vi "Initialize.vi"(8 "error in (no error)":errorcluster, 11 "Function in":refnum<class "Function.lvclass">) -> (0 "error out":errorcluster, 3 "Function out":refnum<class "Function.lvclass">)   [LabVIEW 2016, in "Function Actor.lvlib" / "Function.lvclass"]
doc: "Override configure.vi to setup any parameters for a function before acquiring.\n\nConfigure.vi is called by the 'Initialize Function Actor Core.vi,' which executes before Actor Core of the root function class. The root configure method populates the basic Function UI with information such as the hardware device in use and the name of the function. The base configure method calls 'Acquire.vi' once execution is complete. If beginning a recurring acquisition, it reset the iteration count to zero."
uses:
  <userlib>/Common Components/Function Actor/Function.lvclass
  C:/Program Files (x86)/National Instruments/LabVIEW 2016/vi.lib/ActorFramework/Actor/Actor.lvclass
  <vilib>/ActorFramework/Actor/Actor.lvclass/Actor.ctl
  <vilib>/ActorFramework/Message Enqueuer/Message Enqueuer.lvclass/Message Enqueuer.ctl
  <userlib>/Common Components/Function Actor/Function.lvclass/Function.ctl
  <userlib>/Common Components/Function Messages/Log in MsgList Msg/Log in MsgList Msg.lvclass/Log in MsgList Msg.ctl
  <vilib>/ActorFramework/Message Enqueuer/Init from Existing Queue.vi
  <vilib>/ActorFramework/Message Enqueuer/Enqueue.vi
  <userlib>/Common Components/Function Messages/TCP Connect Msg/TCP Connect Msg.lvclass
  C:/Program Files (x86)/National Instruments/LabVIEW 2016/vi.lib/ActorFramework/Message/Message.lvclass
  <userlib>/Common Components/Function Messages/WebSocket Handshake Msg/WebSocket Handshake Msg.lvclass
  <userlib>/Common Components/Function Messages/Log in MsgList Msg/Log in MsgList Msg.lvclass
  <userlib>/Common Components/Function Actor/Messages/Acquire Msg/Core Iterate Msg.lvclass
  <vilib>/ActorFramework/Message Priority Queue/Priority Enqueue.vi
  <vilib>/ActorFramework/Message Enqueuer/Message Enqueuer.lvclass
  <userlib>/Common Components/Hardware/Abstract Hardware/Hardware.lvclass
  <vilib>/ActorFramework/Actor/Actor.lvclass
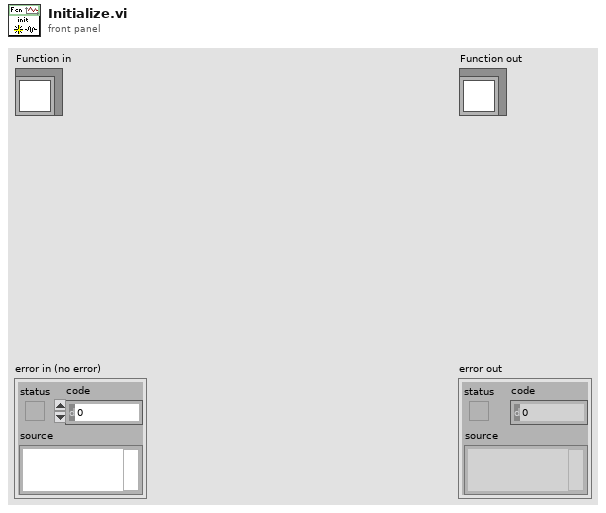
[diagram p1: front panel]
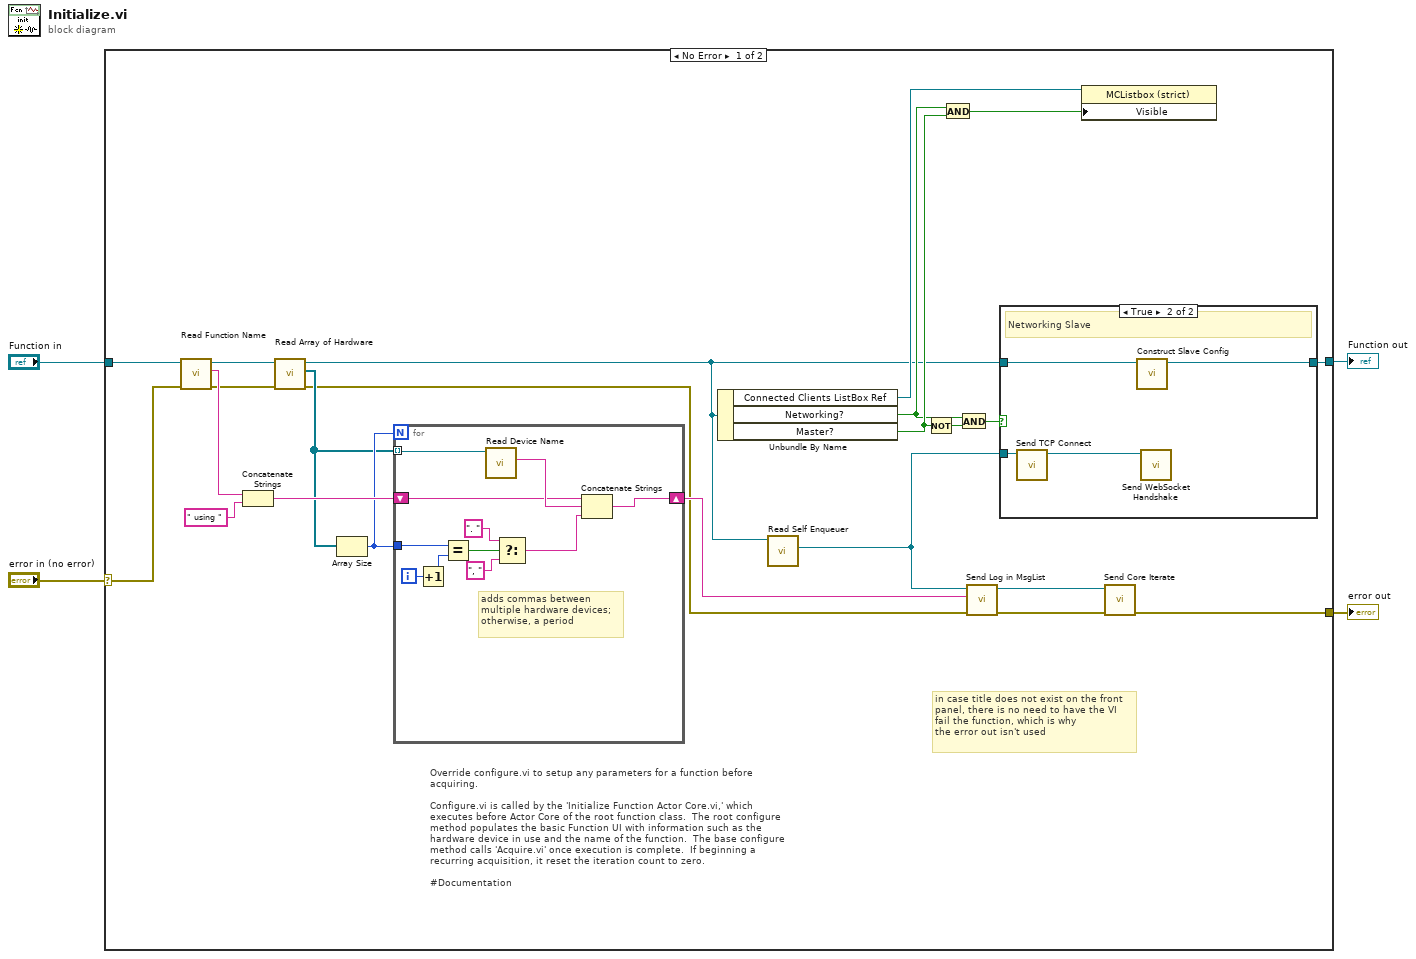
[diagram p0: block diagram]
diagram:
  n1 = case shown="No Error" "error in (no error)" {
    selector: "error in (no error)" -> [w22 w45]
    tunnel: [w15 w45] -> w1
    tunnel: [w11 w44] -> w2
    tunnel: "Function in" -> [w27 w44]
    frame No Error {
      # "Override configure.vi to setup any parameters for a function before acquiring.\n\nConfigure.vi is called by the 'Initialize Function Actor Core.vi,' which executes before Actor Core of the root function class.  The root configure method populates the basic Function UI with information such as the hardware device in use and the name of the function.  The base configure method calls 'Acquire.vi' once execution is complete.  If beginning a recurring acquisition, it reset the iteration count to zero.\n\n#Documentation"
      # "in case title does not exist on the front\npanel, there is no need to have the VI\nfail the function, which is why\nthe error out isn't used"
      n2 = call <userlib>:"Read Function Name.vi"("error in (no error)"=w22, "Function in"=w27) -> ("error out"=w23:errorcluster, "Function Name"=w24:string, "Function out"=w26:refnum<class "Function.lvclass">)  [unwired: 7 in]
      n3 = Concatenate Strings(w24, " using " ("string")) -> (w21:string)
      n4 = call <userlib>:"Read Array of Hardware.vi"("error in (no error)"=w23, "Function in"=w26) -> ("error out"=w16:errorcluster, "Array of Hardware"=w19:refnum<class "Hardware.lvclass">[], "Function out"=w5:refnum<class "Function.lvclass">)  [unwired: 7 in]
      n5 = Array Size(array=w19) -> (size(s)=w20:i32)
      n6 = for {
        N: w20 -> [_]
        tunnel: w19 -> [w43] mode=indexing
        shift-right: [w42] -> w17
        shift-left: w21 -> [w33]
        tunnel: w20 -> [w39]
        i -> [w34]
        # "adds commas between\nmultiple hardware devices;\notherwise, a period"
        n7 = Increment(x=w34) -> (x+1=w40:i32)
        n8 = Equal?(x=w39, y=w40) -> (x = y?=w38:bool)
        n9 = call <userlib>:"Read Device Name.vi"("Analog in"=w43) -> ("Device Name"=w41:string)  [unwired: 8 in, 2 out]
        n10 = Select(t=". " ("string"), s=w38, f=", " ("string")) -> (s? t:f=w37:string)
        n11 = Concatenate Strings(w33, w41, w37) -> (w42:string)
      }
      n12 = Unbundle By Name(w5) -> ("Connected Clients ListBox Ref"=w10:refnum<vi>, "Networking?"=w7:bool, "Master?"=w8:bool)
      n13 = call <vilib>:"Read Self Enqueuer.vi"("Actor"=w5) -> ("Self Enqueuer"=w13:refnum<class "Message Enqueuer.lvclass">)  [unwired: 10 in]
      n14 = Not(x=w8) -> (.not. x?=w12:bool)
      n15 = And(x=w7, y=w8) -> (x .and. y?=w6:bool)
      n16 = And(x=w7, y=w12) -> (x .and. y?=w9:bool)
      n17 = call <userlib>:"Send Log in MsgList.vi"("error in (no error)"=w16, "Msg"=w17, "Message Enqueuer"=w13) -> ("error out"=w18:errorcluster, "Message Enqueuer out"=w14:refnum<class "Message Enqueuer.lvclass">)  [unwired: 7 in]
      n18 = case shown="True" w9 {
        tunnel: w13 -> [_ w32]
        tunnel: w5 -> [w28 w30]
        tunnel: [w28 w29] -> w11
        frame False {
        }
        frame True {
          # "Networking Slave"
          n19 = call <userlib>:"Send TCP Connect.vi"("Message Enqueuer"=w32) -> ("Message Enqueuer out"=w31:refnum<class "Message Enqueuer.lvclass">)  [unwired: 9 in, 1 out]
          n20 = call <userlib>:"Construct Slave Config.vi"("Function in"=w30) -> ("Function out"=w29:refnum<class "Function.lvclass">)  [unwired: 9 in, 1 out]
          n21 = call <userlib>:"Send WebSocket Handshake.vi"("Message Enqueuer"=w31) -> ()  [unwired: 9 in, 2 out]
        }
      }
      n22 = property class="MCListbox (strict)"(reference=w10, "Visible"=w6) -> ()  [unwired: 1 in, 2 out]
      n23 = call <userlib>:"Send Core Iterate.vi"("error in (no error)"=w18, "Message Enqueuer in"=w14) -> ("error out"=w15:errorcluster)  [unwired: 8 in, 1 out]
    }
    frame Error {
    }
  }
  "error out" <- w1
  "Function out" <- w2
